vi "MFCclient.vi"(9 "Setpoint":dbl(slide) max=100.0 step=10.0 scale=0.0..100.0, 10 "Valve":bool, 11 "MFCbasename":string) -> ()   [LabVIEW 2020]
panel:
  out "SPComments":string
  out "ValveComments":string
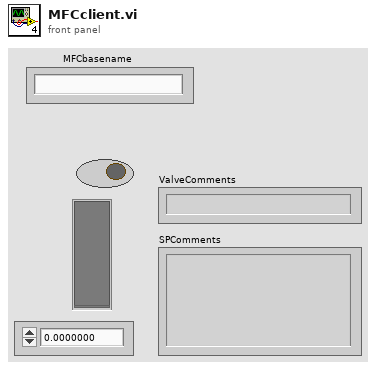
[diagram p1: front panel]
types:
  T1 = typedef "Ch_description_ADAM.ctl" = cluster{"Ch Name":string, "Type":T2, "Function":T3, "Ch State":T4, "Calibration type":T5, "A":dbl, "B":dbl, "C":dbl, "D":dbl, "Comments":string, "Address":T6, "String":string, "Duty":u16}
  T2 = typedef "Module_type_ADAM.ctl" = string
  T3 = typedef "Function_ADAM.ctl" = enum16{"Analogue Input", "Digital Input", "Event counter", "Event rate", "Analogue Output", "Digital Output", "Relay Output"}
  T4 = typedef "Channel_State.ctl" = enum16{"On", "Off", "Always On", "Always Off"}
  T5 = typedef "Calib_type_ADAM.ctl" = string
  T6 = typedef "Address.ctl" = cluster{"Main":i32, "Ch.":i32, "Sub":i32, "Port Name":string}
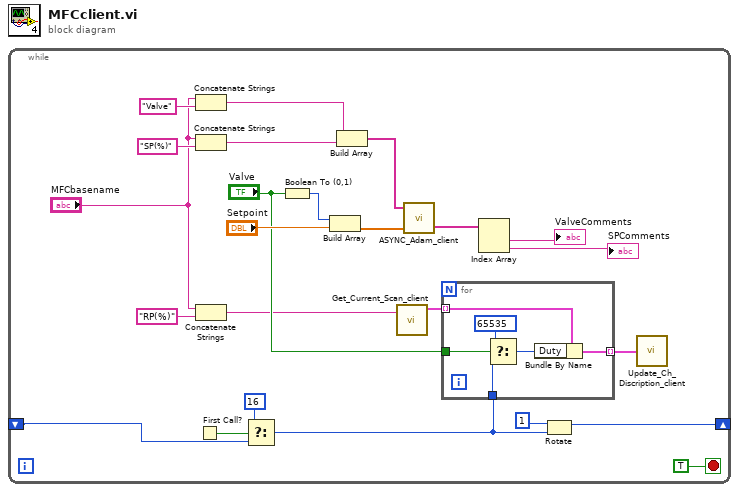
[diagram p0: block diagram]
diagram:
  n1 = while {
    shift-right: [w8] -> _
    shift-left: _ -> [w5]
    stop <- TRUE stop-if-true
    n2 = First Call?() -> (First Call?: T/F=w6:bool)
    n3 = Concatenate Strings("MFCbasename", "Valve" ("string")) -> (w9:string)
    n4 = Concatenate Strings("MFCbasename", "SP(%)" ("string")) -> (w10:string)
    n5 = Concatenate Strings("MFCbasename", "RP(%)" ("string")) -> (w1:string)
    n6 = Select(t=u16 16, s=w6, f=w5) -> (s? t:f=w4:u16)
    n7 = Boolean To (0,1)(Boolean="Valve") -> (0, 1=w22:i16)
    n8 = Build Array(w22, "Setpoint") -> (w24:dbl[])
    n9 = Build Array(w9, w10) -> (w23:string[])
    n10 = call "Get_Current_Scan_client.vi"("singleChannel"=w1) -> ("Ch Description Array"=w17:T1[])  [unwired: 2 in, 2 out]
    n11 = call "ASYNC_Adam_client.vi"("Values"=w24, "Channel Names"=w23) -> ("Scan Comments"=w20:string[])  [unwired: 1 in, 1 out]
    n12 = for {
      tunnel: w17 -> [w30] mode=indexing
      tunnel: [w29] -> w16 mode=indexing
      tunnel: "Valve" -> [w27]
      tunnel: w4 -> [w25]
      n13 = Select(t=u16 65535 ("Duty"), s=w27, f=w25) -> (s? t:f=w26:u16)
      n14 = Bundle By Name(cluster=w30, "Duty"=w26) -> (w29:T1)
    }
    n15 = Index Array(array=w20) -> (element #1=→"ValveComments":string, element #2=→"SPComments":string)  [unwired: 2 in]
    n16 = Rotate(1:w4, 2:u16 1 ("f")) -> (0:w8:u16)
    n17 = call "Update_Ch_Discription_client.vi"("Channels to update In"=w16) -> ()  [unwired: 1 out]
  }
